vi "NXT Camera Test7.vi"() -> ()   [LabVIEW 2016]
uses:
  <vilib>/NXT/Block Support/NXT_InputPort.ctl
  <vilib>/NXT/Block Support/NXT_OutputPort.ctl
  <vilib>/NXT/NXTIO Xnodes/NXTIONodeSubVIs/NXTMoveMotors.vi
  <vilib>/NXT/NXTIO Xnodes/NXTIONodeSubVIs/NXTStopMotors.vi
  <vilib>/NXT/Dual Mode Library/Waits/Wait_Num.vi
  <vilib>/NXT/Subs/LVHSConnector.ctl
  <vilib>/NXT/NXTIO Xnodes/AddressXNode/NXTIOAddress.xnode
  <vilib>/NXT/NXTIO Xnodes/NXTIOXNode/NXTIO.xnode
  <vilib>/NXT/LegoClasses/BrickReference/BrickReference.lvclass
panel:
  out "Power":bool
  out "X Upper Left":u8
  out "X Lower Right":u8
  out "Y Lower Right":u8
  out "Y Upper Left":u8
  out "Count":u8
  out "Color":u8
  in  "Cluster":T1 {"Tracking Mode" items=["Disable Tracking", "Get First Object", "Get n th Object", "Enable Tracking", "Sort Objects  by size", "Sort Objects  by Colors", "Illumination on ", "Illumination Off", "Write Colormap", "Read Colormap", "Line tracking mode", "Object Tracking mode"]}
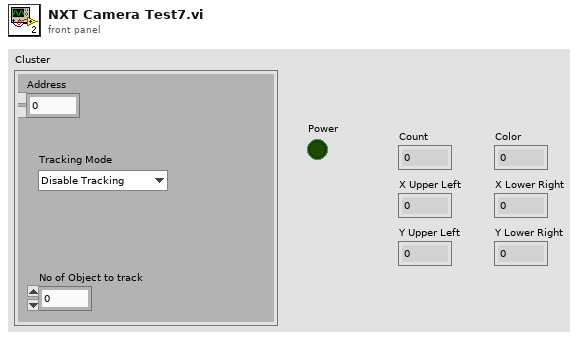
[diagram p1: front panel]
types:
  T1 = cluster{"Address":dbl, "No of Object to track":dbl, "Tracking Mode":u8}
  T2 = cluster{"Tracking Mode":u8, "Object Number to Track":u8, "Address":u8}
  T3 = typedef "NXT_InputPort.ctl" = u32
  T4 = typedef "LVHSConnector.ctl" = refnum<class "BrickReference.lvclass">
  T5 = cluster{"Total Tracked Objects":u8, "Color":u8, "X Upper Left":u8, "Y Upper Left":u8, "X Lower Right":u8, "Y Lower Right":u8, "Status (boolean)":bool}
  T6 = typedef "NXT_OutputPort.ctl" = u8
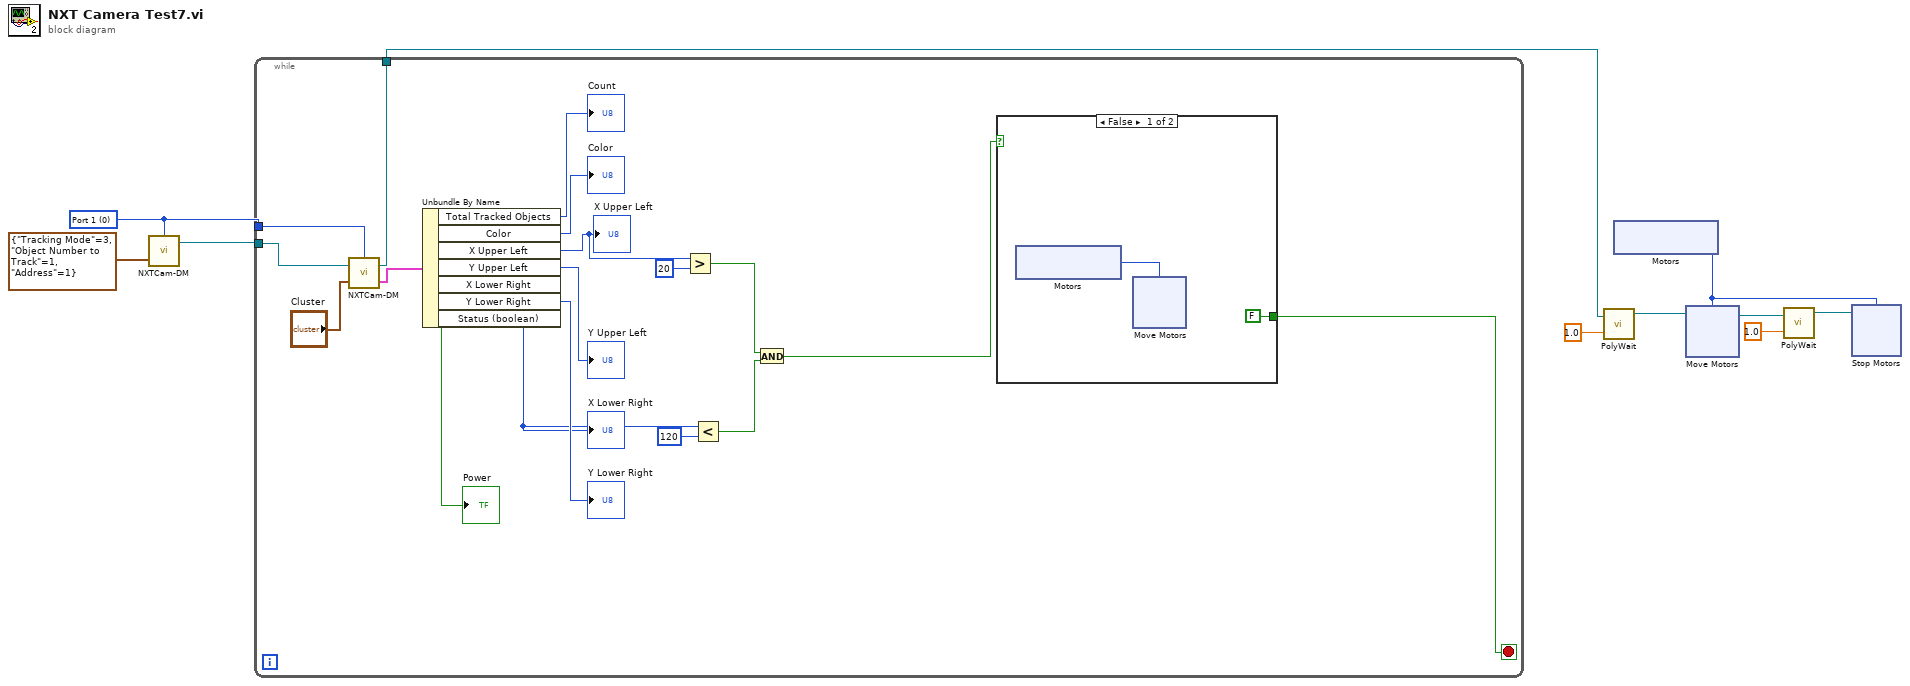
[diagram p0: block diagram]
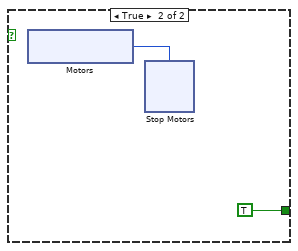
[diagram p2: hidden frame]
diagram:
  w9 = T3 0 items=["Port 1", "Port 2", "Port 3", "Port 4"] ("Input Port")
  n1 = call "NXTCam-DM.vi"("Input of NXTCam"=T2 {"Tracking Mode"=3, "Object Number to Track"=1, "Address"=1}, "Input Port"=w9) -> ("NXT dup"=w8:T4)  [unwired: 1 in, 1 out]
  n2 = while {
    tunnel: w9 -> [w26]
    tunnel: w8 -> [w25]
    tunnel: [w11] -> w1
    stop <- w12 stop-if-true
    n3 = call "NXTCam-DM.vi"("Input of NXTCam"="Cluster", "NXT"=w25, "Input Port"=w26) -> ("Output of NXTCam"=w21:T5, "NXT dup"=w11:T4)
    n4 = Unbundle By Name(w21) -> ("Total Tracked Objects"=→"Count":u8, "Color"=→"Color":u8, "X Upper Left"=w19:u8, "Y Upper Left"=→"Y Upper Left":u8, "X Lower Right"=w17:u8, "Y Lower Right"=→"Y Lower Right":u8, "Status (boolean)"=→"Power":bool)
    "X Upper Left" <- w19
    "X Lower Right" <- w17
    n5 = Greater?(x=w19, y=u8 20) -> (0:w15:bool)
    n6 = Less?(x=w17, y=u8 120) -> (x < y?=w14:bool)
    n7 = And(x=w15, y=w14) -> (x .and. y?=w13:bool)
    n8 = case shown="False" w13 {
      tunnel: [FALSE TRUE] -> w12
      frame False {
        n9 = xnode "Motors"() -> ("Motor"=w30:T6)
        n10 = xnode "Move Motors"("Motors"=w30) -> ()  [unwired: 2 in, 1 out]
      }
      frame True {
        n11 = xnode "Motors"() -> ("Motor"=w40:T6)
        n12 = xnode "Stop Motors"("Motors"=w40) -> ()  [unwired: 1 in, 1 out]
      }
    }
  }
  n13 = call-poly <vilib>:"PolyWait.vi"("Time (1 sec)"=sgl 1.0, "NXT/EV3"=w1) -> ("NXT/EV3"=w6:T4)  [unwired: 2 in]
  n14 = xnode "Motors"() -> ("Motor"=w2:T6)
  n15 = xnode "Move Motors"("Motors"=w2, "NXT/EV3"=w6) -> ("NXT/EV3"=w5:T4)  [unwired: 1 in]
  n16 = call-poly <vilib>:"PolyWait.vi"("Time (1 sec)"=sgl 1.0, "NXT/EV3"=w5) -> ("NXT/EV3"=w3:T4)  [unwired: 2 in]
  n17 = xnode "Stop Motors"("Motors"=w2, "NXT/EV3"=w3) -> ()  [unwired: 1 out]
